vi "Curtin_BoxCar2.vi"(0 "Original Data":waveform(dbl)(graph), 1 "Cutoff (sec)":dbl=0.1) -> (3 "Cutoff Data":waveform(dbl)(graph))   [LabVIEW 2022 SP3]
panel:
  out "Cutoff Data 2":waveform(dbl)[](graph)
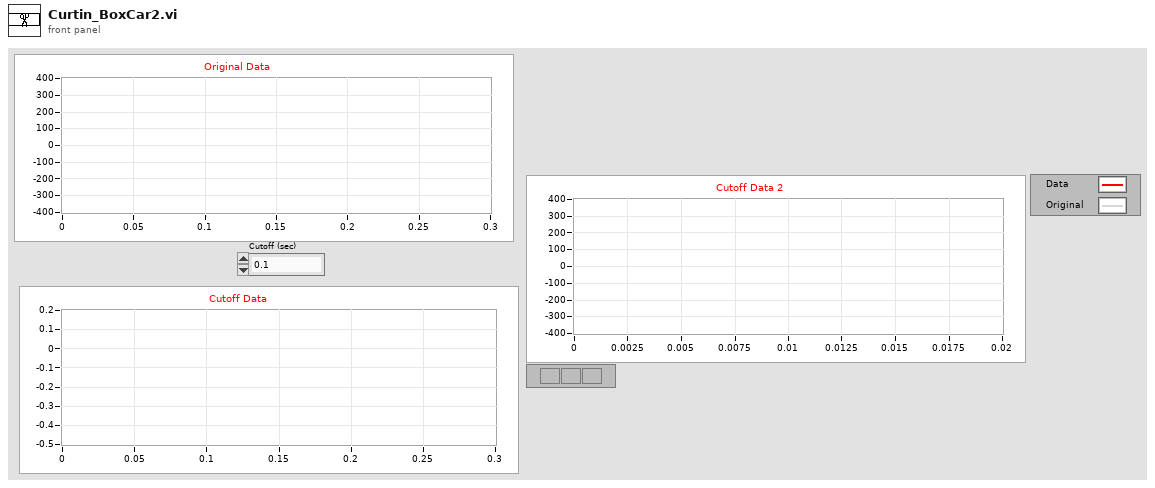
[diagram p1: front panel]
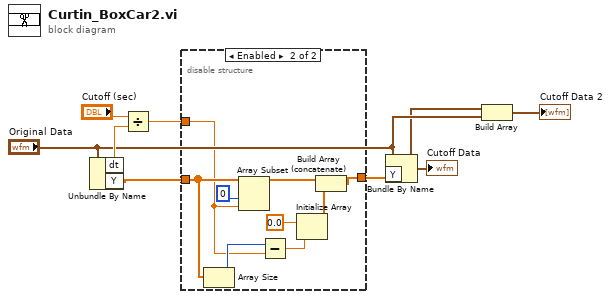
[diagram p0: block diagram]
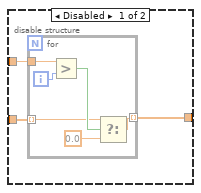
[diagram p2: hidden frame]
diagram:
  n1 = Unbundle By Name("Original Data") -> ("dt"=w7:dbl, "Y"=w3:dbl[])
  n2 = Divide(x="Cutoff (sec)", y=w7) -> (x/y=w5:dbl)
  n3 = disable-structure shown="Enabled" {
    disable-tunnel: [w11 w19] -> w4
    disable-tunnel: w5 -> [w10 w23]
    disable-tunnel: w3 -> [w9 w26]
    frame Disabled {
      n4 = for {
        tunnel: w10 -> [w16]
        tunnel: w9 -> [w14] mode=indexing
        tunnel: [w13] -> w11 mode=indexing
        i -> [w17]
        n5 = Greater?(x=w16, y=w17) -> (0:w15:bool)
        n6 = Select(t=w14, s=w15, f=0.0) -> (s? t:f=w13:dbl)
      }
    }
    frame Enabled {
      n7 = Array Size(array=w26) -> (size(s)=w24:i32)
      n8 = Array Subset(array=w26, index=0, length=w23) -> (w21:dbl[])
      n9 = Subtract(x=w24, y=w23) -> (x-y=w22:dbl)
      n10 = Initialize Array(0.0, w22) -> (w20:dbl[])
      n11 = Build Array (concatenate)(w21, w20) -> (w19:dbl[])
    }
  }
  n12 = Bundle By Name(cluster="Original Data", "Y"=w4) -> (w1:waveform(dbl))
  "Cutoff Data" <- w1
  n13 = Build Array(w1, "Original Data") -> (→"Cutoff Data 2":waveform(dbl)[])
